vi "String_Hex String to readable text.vi"(4 "Hex string":string) -> (1 "Readable Hex":string)   [LabVIEW 2020]
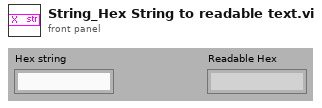
[diagram p1: front panel]
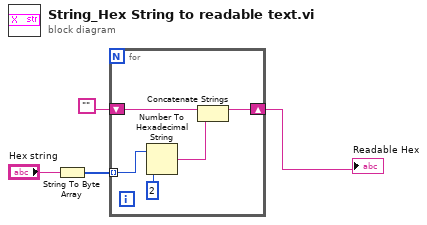
[diagram p0: block diagram]
diagram:
  n1 = String To Byte Array(string="Hex string") -> (unsigned byte array=w3:u8[])
  n2 = for {
    tunnel: w3 -> [w9] mode=indexing
    shift-right: [w7] -> w1
    shift-left: "" -> [w8]
    n3 = Number To Hexadecimal String(1:i16 2 ("width (-)"), 2:w9) -> (0:w6:string)
    n4 = Concatenate Strings(w8, w6) -> (w7:string)
  }
  "Readable Hex" <- w1
